vi "Array Get Long Array.vi"(8 "error in (no error)":errorcluster, 11 "Array DVR in":refnum<data-value>) -> (0 "error out":errorcluster, 1 "Array dimensions":i32[](array[numeric]), 2 "I64 array out":i64[](array[numeric]), 3 "Array DVR out":refnum<data-value>)   [LabVIEW 2015, in "MDSplus.lvlib"]
uses:
  <vilib>/MDSplus/Library/MDSplus.lvlib
  <vilib>/MDSplus/Classes/Data_Class/Array_Class/Array.lvclass
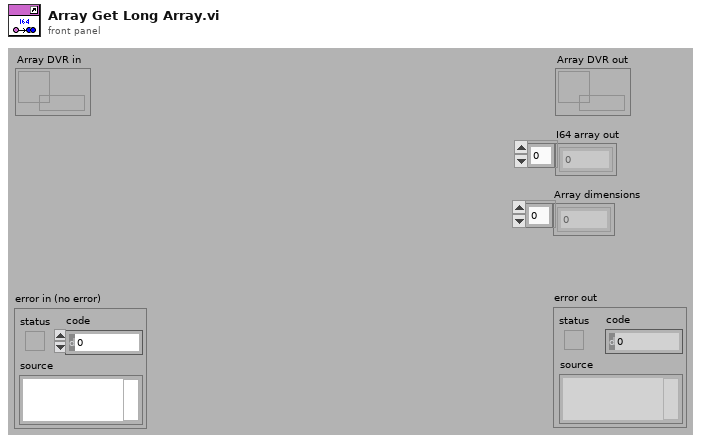
[diagram p1: front panel]
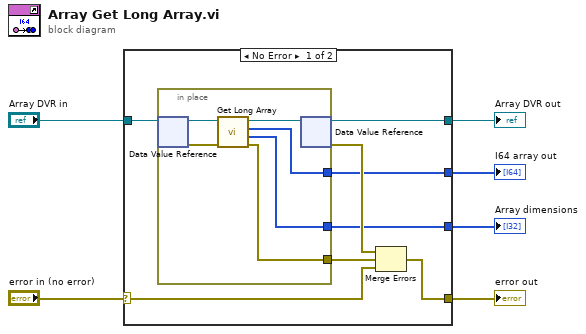
[diagram p0: block diagram]
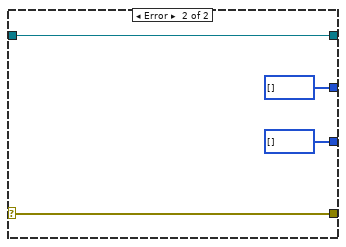
[diagram p2: hidden frame]
diagram:
  n1 = case shown="No Error" "error in (no error)" {
    selector: "error in (no error)" -> [w12 w24]
    tunnel: "Array DVR in" -> [w14 w23]
    tunnel: [w10 w24] -> w6
    tunnel: [w9 w23] -> w3
    tunnel: [w8 i64[] [] ("SGL array out")] -> w2
    tunnel: [w7 i32[] [] ("Array dimensions")] -> w1
    frame No Error {
      n2 = in-place {
        in-place-border: [w18] -> w13
        in-place-border: [w16] -> w8
        in-place-border: [w15] -> w7
        n3 = in-place-dvr #1(w14) -> (w20:refnum<class "Array.lvclass">, w17:errorcluster)
        n4 = call-dynamic "Get Long Array.vi"("error in (no error)"=w17, "Array in"=w20) -> ("error out"=w18:errorcluster, "Array dimensions"=w15:i32[], "I64 array out"=w16:i64[], "Array out"=w19:refnum<class "Array.lvclass">)  [unwired: 6 in]
        n5 = in-place-dvr #1(w19) -> (w9:refnum<data-value>, w11:errorcluster)
      }
      n6 = Merge Errors(w11, w13, w12) -> (w10:errorcluster)
    }
    frame Error {
    }
  }
  "error out" <- w6
  "Array DVR out" <- w3
  "I64 array out" <- w2
  "Array dimensions" <- w1
